vi "Destroy HTTP Session.vi"(8 "error in (no error)":errorcluster, 11 "http-client in":refnum<class "httpClient.lvclass">) -> (0 "error out":errorcluster, 3 "http-client out":refnum<class "httpClient.lvclass">)   [LabVIEW 2020, in "httpClient.lvlib" / "httpClient.lvclass"]
uses:
  httpClient.lvclass
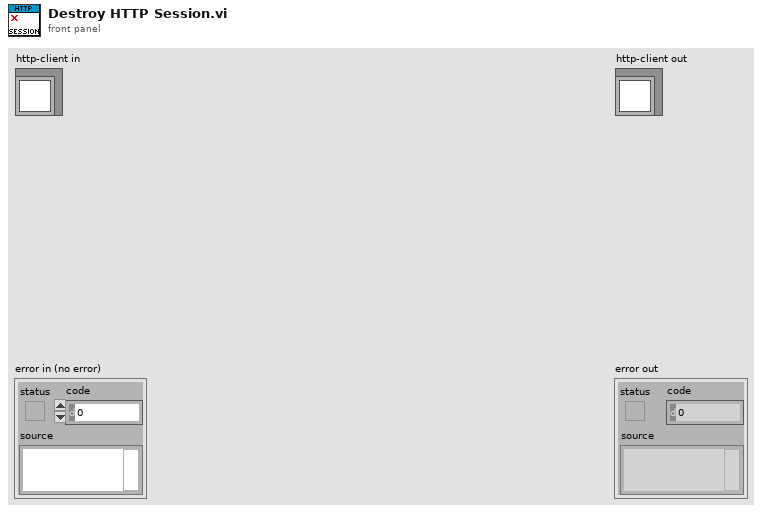
[diagram p1: front panel]
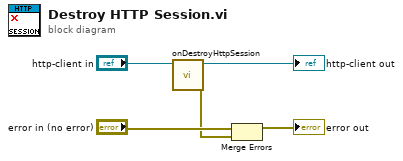
[diagram p0: block diagram]
diagram:
  n1 = call-dynamic "onDestroyHttpSession.vi"("http-client in"="http-client in") -> ("error out"=w2:errorcluster, "http-client out"=→"http-client out":refnum<class "httpClient.lvclass">)  [unwired: 9 in]
  n2 = Merge Errors("error in (no error)", w2) -> (→"error out":errorcluster)
